vi "仁科空调控制器告警存储.vi"   [LabVIEW 2016, in "环境动力监测库.lvlib" / "空调库.lvlib"]
uses:
  <vilib>/ptbypt/NI_PtbyPt.lvlib
types:
  T1 = cluster{"时间标识":timestamp, "设备":string, "日志信息":string}
  T2 = cluster{"温湿度解析":cluster{"湿度":dbl, "温度":dbl}, "传感器状态输出":cluster{"第一路电流A":u16, "第二路电流A":u16, "空调控制模式":enum16{"远程", "自动"}, "蜂鸣器和继电器报警输出状态":enum16{"正常", "报警"}, "秒数高16位":u16, "秒数低16位":u16}, "告警状态":cluster{"第一路开关机失败":bool, "第二路开关机失败":bool, "温度超上限报警":bool, "温度超下限报警":bool}, "运行状态":cluster{"第一路空调运行状态":enum16{"停止", "制冷", "制热", "未知"}, "第二路空调运行状态":enum16{"停止", "制冷", "制热", "未知"}}}
  T3 = cluster{"漏水监测输出":cluster{"漏水监测告警":bool, "告警内容":string}, "门禁监测输出":cluster{"门禁监测告警":bool, "告警内容":string}, "门禁监测输出2":cluster{"门禁监测告警":bool, "告警内容":string}, "温湿度监测输出":cluster{"温湿度监测告警":bool, "告警内容":string}, "烟雾监测输出":cluster{"烟雾监测告警":bool, "告警内容":string}, "空调监测输出":cluster{"空调监测告警":bool, "告警内容":string}, "自动重合闸输出":cluster{"自动重合闸告警":bool, "告警内容":string}, "红外入侵输出":cluster{"红外入侵告警":bool, "告警内容":string}, "振动输出":cluster{"振动告警":bool, "告警内容":string}, "UPS输出":cluster{"UPS告警":bool, "告警内容":string}, "蓄电池输出":cluster{"蓄电池告警":bool, "告警内容":string}, "蓄电池输出2":cluster{"蓄电池告警":bool, "告警内容":string}, "GPS输出":cluster{"定位告警":bool, "告警内容":string}, "北斗输出":cluster{"定位告警":bool, "告警内容":string}, "气象输出":cluster{"气象告警":bool, "告警内容":string}}
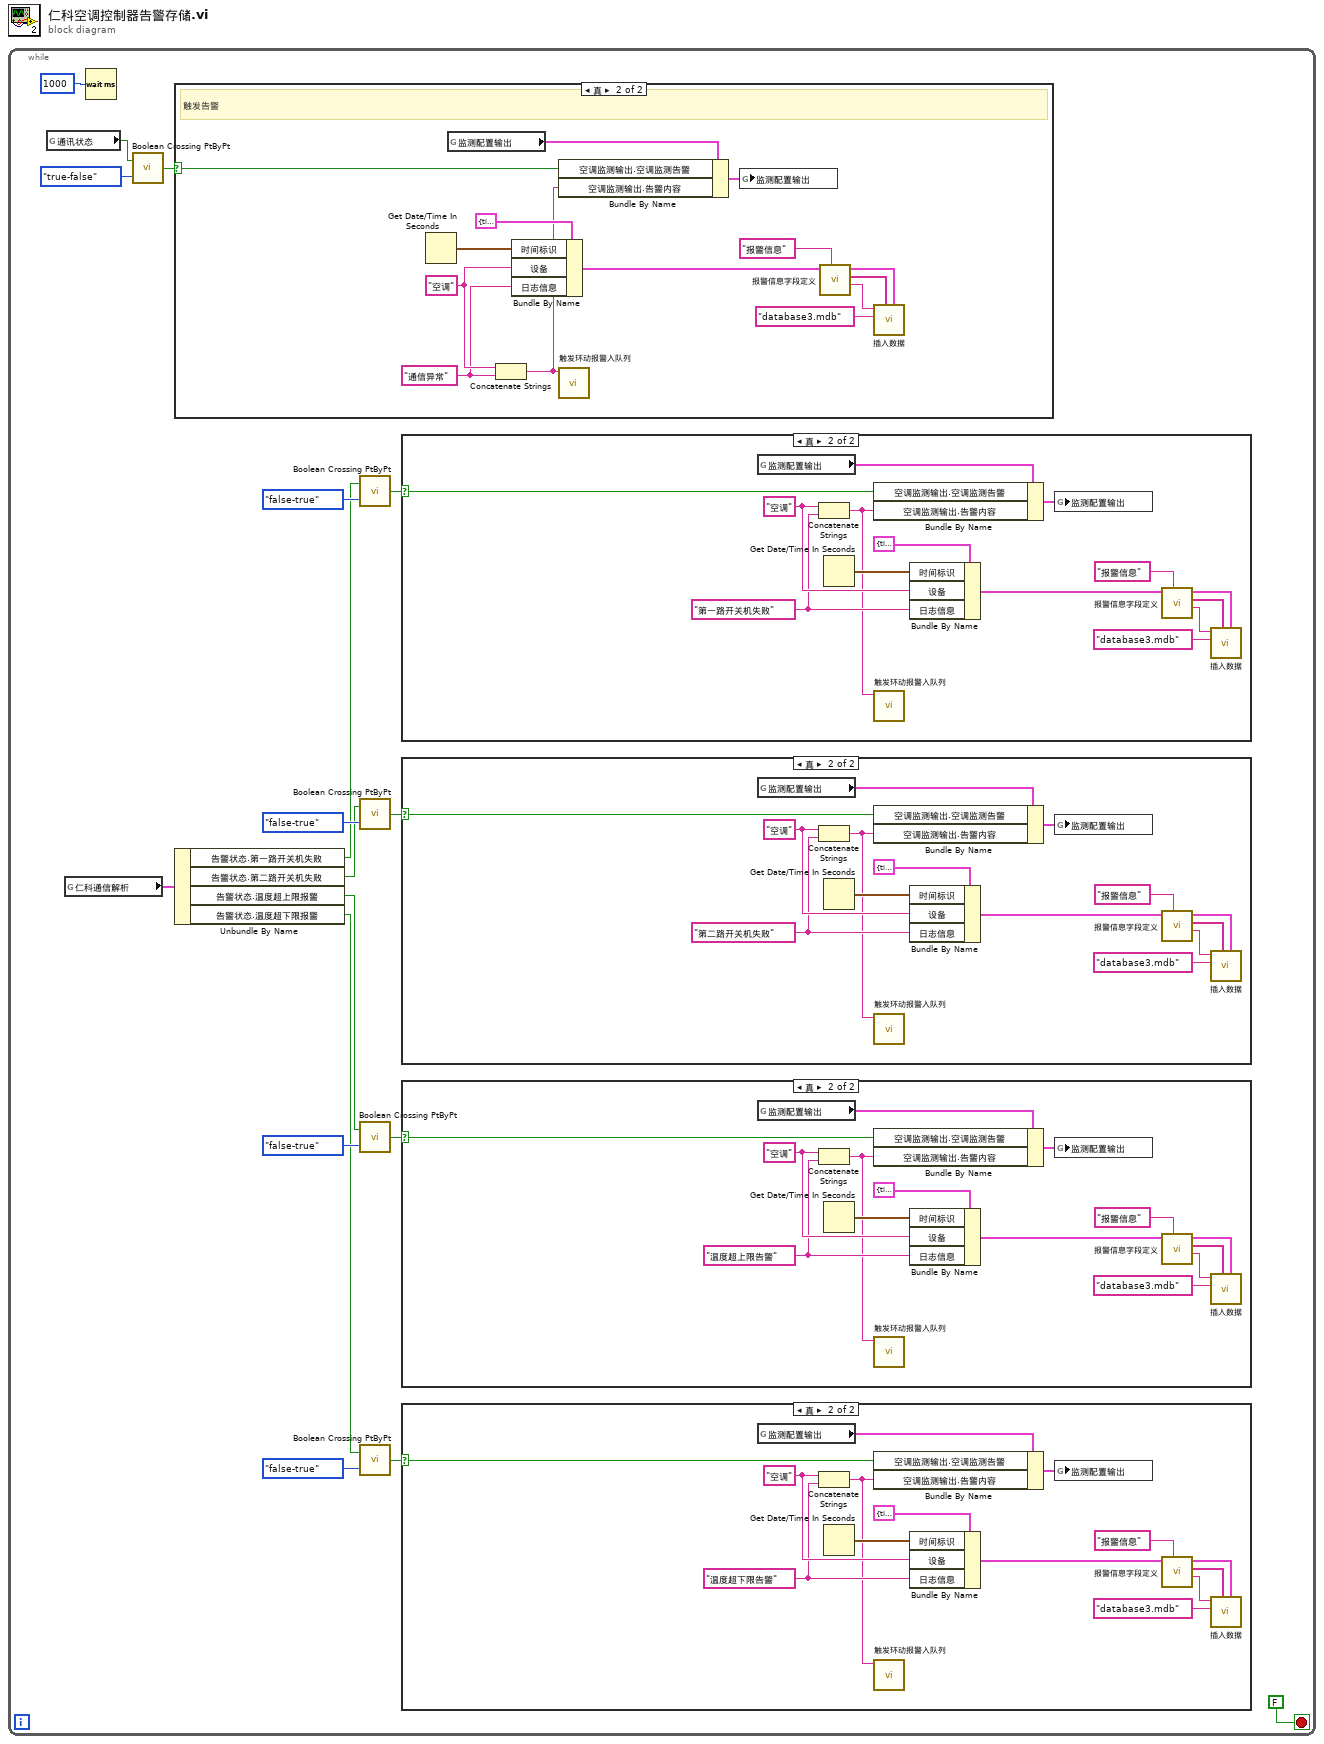
[diagram p0: block diagram]
diagram:
  n1 = while {
    stop <- FALSE stop-if-true
    n2 = global read "断电保存全局变量.vi" "通讯状态"() -> (w6:bool)
    n3 = global read "内部交互全局变量.vi" "仁科通信解析"() -> (w5:T2)
    n4 = Wait (ms)(milliseconds to wait=u32 1000 ("等待时间（毫秒）")) -> ()  [unwired: 1 out]
    n5 = call <vilib>:"Boolean Crossing PtByPt.vi"("direction"=enum16{"either", "false-true", "true-false"}."true-false", "input"=w6) -> ("crossing"=w15:bool)  [unwired: 1 in]
    n6 = case shown="真" w15 {
      selector: w15 -> [_ w75]
      frame False {
      }
      frame True {
        w77 = "通信异常" ("日志信息")
        w78 = "空调" ("设备")
        # "触发告警"
        n7 = Get Date/Time In Seconds() -> (seconds since 1Jan1904=w88:timestamp)
        n8 = global read "断电保存全局变量.vi" "监测配置输出"() -> (w79:T3)
        n9 = Concatenate Strings(w78, w77) -> (w76:string)
        n10 = Bundle By Name(cluster=T1 {"时间标识"=timestamp(0 s since 1904-01-01), "设备"="", "日志信息"=""} ("data in"), "时间标识"=w88, "设备"=w78, "日志信息"=w77) -> (w87:T1)
        n11 = Bundle By Name(cluster=w79, "空调监测输出.空调监测告警"=w75, "空调监测输出.告警内容"=w76) -> (w80:T3)
        n12 = call "触发环动报警入队列.vi"("报警内容"=w76) -> ()  [unwired: 11 in]
        n13 = global write "断电保存全局变量.vi" "监测配置输出"(w80) -> ()
        n14 = call "报警信息字段定义.vi"("table输入"="报警信息", "data in"=w87) -> ("table输出"=w83:string, "columns"=w82:string[], "data out"=w81:T1)  [unwired: 7 in]
        n15 = call "插入数据.vi"("data"=w81, "columns"=w82, "database"="database3.mdb", "table"=w83) -> ()  [unwired: 7 in, 1 out]
      }
    }
    n16 = Unbundle By Name(w5) -> ("告警状态.第一路开关机失败"=w3:bool, "告警状态.第二路开关机失败"=w2:bool, "告警状态.温度超上限报警"=w4:bool, "告警状态.温度超下限报警"=w1:bool)
    n17 = call <vilib>:"Boolean Crossing PtByPt.vi"("direction"=enum16{"either", "false-true", "true-false"}."false-true", "input"=w3) -> ("crossing"=w11:bool)  [unwired: 1 in]
    n18 = call <vilib>:"Boolean Crossing PtByPt.vi"("direction"=enum16{"either", "false-true", "true-false"}."false-true", "input"=w2) -> ("crossing"=w9:bool)  [unwired: 1 in]
    n19 = call <vilib>:"Boolean Crossing PtByPt.vi"("direction"=enum16{"either", "false-true", "true-false"}."false-true", "input"=w4) -> ("crossing"=w13:bool)  [unwired: 1 in]
    n20 = call <vilib>:"Boolean Crossing PtByPt.vi"("direction"=enum16{"either", "false-true", "true-false"}."false-true", "input"=w1) -> ("crossing"=w7:bool)  [unwired: 1 in]
    n21 = case shown="真" w11 {
      selector: w11 -> [_ w50]
      frame False {
      }
      frame True {
        w48 = "第一路开关机失败" ("日志信息")
        w49 = "空调" ("设备")
        n22 = global read "断电保存全局变量.vi" "监测配置输出"() -> (w51:T3)
        n23 = Concatenate Strings(w49, w48) -> (w47:string)
        n24 = Get Date/Time In Seconds() -> (seconds since 1Jan1904=w60:timestamp)
        n25 = Bundle By Name(cluster=w51, "空调监测输出.空调监测告警"=w50, "空调监测输出.告警内容"=w47) -> (w52:T3)
        n26 = call "触发环动报警入队列.vi"("报警内容"=w47) -> ()  [unwired: 11 in]
        n27 = Bundle By Name(cluster=T1 {"时间标识"=timestamp(0 s since 1904-01-01), "设备"="", "日志信息"=""} ("data in"), "时间标识"=w60, "设备"=w49, "日志信息"=w48) -> (w59:T1)
        n28 = global write "断电保存全局变量.vi" "监测配置输出"(w52) -> ()
        n29 = call "报警信息字段定义.vi"("table输入"="报警信息", "data in"=w59) -> ("table输出"=w55:string, "columns"=w54:string[], "data out"=w53:T1)  [unwired: 7 in]
        n30 = call "插入数据.vi"("data"=w53, "columns"=w54, "database"="database3.mdb", "table"=w55) -> ()  [unwired: 7 in, 1 out]
      }
    }
    n31 = case shown="真" w9 {
      selector: w9 -> [_ w36]
      frame False {
      }
      frame True {
        w34 = "第二路开关机失败" ("日志信息")
        w35 = "空调" ("设备")
        n32 = global read "断电保存全局变量.vi" "监测配置输出"() -> (w37:T3)
        n33 = Concatenate Strings(w35, w34) -> (w33:string)
        n34 = Get Date/Time In Seconds() -> (seconds since 1Jan1904=w46:timestamp)
        n35 = Bundle By Name(cluster=w37, "空调监测输出.空调监测告警"=w36, "空调监测输出.告警内容"=w33) -> (w38:T3)
        n36 = call "触发环动报警入队列.vi"("报警内容"=w33) -> ()  [unwired: 11 in]
        n37 = Bundle By Name(cluster=T1 {"时间标识"=timestamp(0 s since 1904-01-01), "设备"="", "日志信息"=""} ("data in"), "时间标识"=w46, "设备"=w35, "日志信息"=w34) -> (w45:T1)
        n38 = global write "断电保存全局变量.vi" "监测配置输出"(w38) -> ()
        n39 = call "报警信息字段定义.vi"("table输入"="报警信息", "data in"=w45) -> ("table输出"=w41:string, "columns"=w40:string[], "data out"=w39:T1)  [unwired: 7 in]
        n40 = call "插入数据.vi"("data"=w39, "columns"=w40, "database"="database3.mdb", "table"=w41) -> ()  [unwired: 7 in, 1 out]
      }
    }
    n41 = case shown="真" w13 {
      selector: w13 -> [_ w64]
      frame False {
      }
      frame True {
        w62 = "温度超上限告警" ("日志信息")
        w63 = "空调" ("设备")
        n42 = global read "断电保存全局变量.vi" "监测配置输出"() -> (w65:T3)
        n43 = Concatenate Strings(w63, w62) -> (w61:string)
        n44 = Get Date/Time In Seconds() -> (seconds since 1Jan1904=w74:timestamp)
        n45 = Bundle By Name(cluster=w65, "空调监测输出.空调监测告警"=w64, "空调监测输出.告警内容"=w61) -> (w66:T3)
        n46 = call "触发环动报警入队列.vi"("报警内容"=w61) -> ()  [unwired: 11 in]
        n47 = Bundle By Name(cluster=T1 {"时间标识"=timestamp(0 s since 1904-01-01), "设备"="", "日志信息"=""} ("data in"), "时间标识"=w74, "设备"=w63, "日志信息"=w62) -> (w73:T1)
        n48 = global write "断电保存全局变量.vi" "监测配置输出"(w66) -> ()
        n49 = call "报警信息字段定义.vi"("table输入"="报警信息", "data in"=w73) -> ("table输出"=w69:string, "columns"=w68:string[], "data out"=w67:T1)  [unwired: 7 in]
        n50 = call "插入数据.vi"("data"=w67, "columns"=w68, "database"="database3.mdb", "table"=w69) -> ()  [unwired: 7 in, 1 out]
      }
    }
    n51 = case shown="真" w7 {
      selector: w7 -> [_ w22]
      frame False {
      }
      frame True {
        w20 = "温度超下限告警" ("日志信息")
        w21 = "空调" ("设备")
        n52 = global read "断电保存全局变量.vi" "监测配置输出"() -> (w23:T3)
        n53 = Concatenate Strings(w21, w20) -> (w19:string)
        n54 = Get Date/Time In Seconds() -> (seconds since 1Jan1904=w32:timestamp)
        n55 = Bundle By Name(cluster=w23, "空调监测输出.空调监测告警"=w22, "空调监测输出.告警内容"=w19) -> (w24:T3)
        n56 = call "触发环动报警入队列.vi"("报警内容"=w19) -> ()  [unwired: 11 in]
        n57 = Bundle By Name(cluster=T1 {"时间标识"=timestamp(0 s since 1904-01-01), "设备"="", "日志信息"=""} ("data in"), "时间标识"=w32, "设备"=w21, "日志信息"=w20) -> (w31:T1)
        n58 = global write "断电保存全局变量.vi" "监测配置输出"(w24) -> ()
        n59 = call "报警信息字段定义.vi"("table输入"="报警信息", "data in"=w31) -> ("table输出"=w27:string, "columns"=w26:string[], "data out"=w25:T1)  [unwired: 7 in]
        n60 = call "插入数据.vi"("data"=w25, "columns"=w26, "database"="database3.mdb", "table"=w27) -> ()  [unwired: 7 in, 1 out]
      }
    }
  }
